vi "Sort Tab Parent Info for Children.vi"(8 "Error In":errorcluster, 10 "Additional Labels":string[][](array[string]), 11 "Control Information in":string[][](array[string])) -> (0 "Error Out":errorcluster, 2 "Broken Out Additional Labels":string[][][](array[string]), 3 "Control Info by Page":string[][][](array[string]))   [LabVIEW 2017, in "Localization.lvlib"]
doc: "TAkes the Control Items and Additional Information and sorts the additional information to be added to sub elements. Of a cluster is separates the information of the cluster into the information that gets written into the specific controls of the cluster.\n\nChoose Movement Consulting, LLC"
uses:
  Localization.lvlib
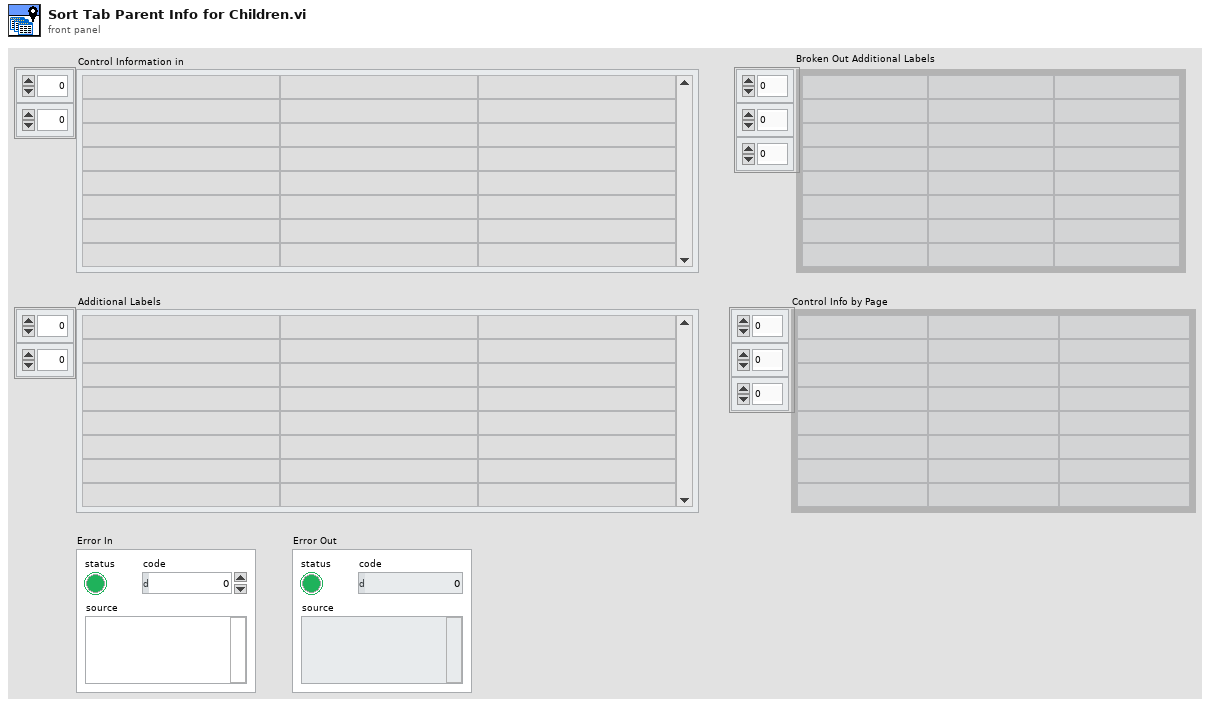
[diagram p1: front panel]
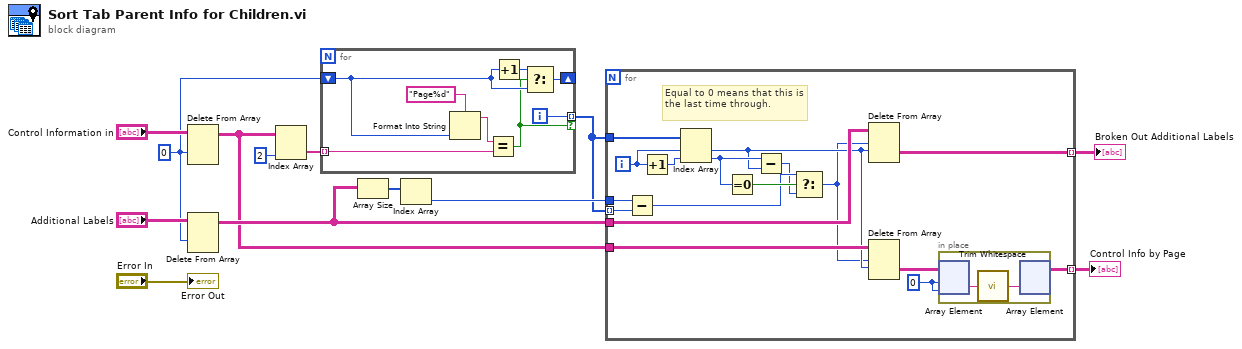
[diagram p0: block diagram]
diagram:
  w3 = 0 ("index (row)")
  n1 = Delete From Array(array="Control Information in", index (row)=w3) -> (array with subset deleted=w1:string[][])  [unwired: 2 in, 1 out]
  n2 = Delete From Array(array="Additional Labels", index (row)=w3) -> (array with subset deleted=w8:string[][])  [unwired: 2 in, 1 out]
  n3 = Index Array(array=w1, index (col)=2 ("disabled index (col)")) -> (element=w4:string[])  [unwired: 1 in]
  n4 = for {
    tunnel: w4 -> [w20] mode=indexing
    shift-right: [w16] -> _
    shift-left: w3 -> [w18]
    tunnel: [w15] -> w2 mode=indexing if=w14
    i -> [w15]
    n5 = Format Into String(format string="Page%d", w18) -> (resulting string=w19:string)  [unwired: 2 in, 1 out]
    n6 = Equal?(x=w19, y=w20) -> (x = y?=w14:bool)
    n7 = Increment(x=w18) -> (x+1=w17:i32)
    n8 = Select(t=w17, s=w14, f=w18) -> (s? t:f=w16:i32)
  }
  n9 = Array Size(array=w8) -> (size(s)=w7:i32[])
  n10 = Index Array(array=w7) -> (element=w6:i32)  [unwired: 1 in]
  n11 = for {
    tunnel: w2 -> [w38]
    tunnel: [w35] -> w9 mode=indexing
    tunnel: w2 -> [w28] mode=indexing
    tunnel: w8 -> [w34]
    tunnel: w6 -> [w31]
    tunnel: [w22] -> w5 mode=indexing
    tunnel: w1 -> [w27]
    i -> [w37]
    w24 = 0
    # "Equal to 0 means that this is the last time through."
    n12 = Subtract(x=w31, y=w28) -> (x-y=w30:i32)
    n13 = Increment(x=w37) -> (x+1=w36:i32)
    n14 = Index Array(array=w38, index #1=w37, index #2=w36) -> (element #1=w26:i32, element #2=w33:i32)
    n15 = Equal To 0?(x=w33) -> (x = 0?=w32:bool)
    n16 = Subtract(x=w33, y=w26) -> (x-y=w29:i32)
    n17 = Select(t=w30, s=w32, f=w29) -> (s? t:f=w25:i32)
    n18 = Delete From Array(array=w34, length=w25, index (row)=w26) -> (deleted portion=w35:string[][])  [unwired: 1 in, 1 out]
    n19 = Delete From Array(array=w27, length=w25, index (row)=w26) -> (deleted portion=w23:string[][])  [unwired: 1 in, 1 out]
    n20 = in-place {
      n21 = in-place-array #1(w23, w24, w24) -> (w40:string)
      n22 = call <vilib>:"Trim Whitespace.vi"("string"=w40) -> ("trimmed string"=w39:string)  [unwired: 1 in]
      n23 = in-place-array #1(w39) -> (w22:string[][])  [unwired: 2 out]
    }
  }
  "Broken Out Additional Labels" <- w9
  "Control Info by Page" <- w5
  "Error Out" <- "Error In"
